vi "Async.Engine.Close.vi"(8 "error in (no error)":errorcluster, 11 "Async in":refnum<class "VS Inline Async API.lvclass">) -> (0 "error out":errorcluster, 3 "Async out":refnum<class "VS Inline Async API.lvclass">)   [LabVIEW 2015, in "VS Inline Async API.lvlib" / "VS Inline Async API.lvclass"]
uses:
  VS Inline Async API.lvclass
  VS Inline Async API.lvclass/VS Inline Async API.ctl
  <vilib>/NI Veristand/Custom Device Tools/Custom Device Utility Library/NI VeriStand - Print Debug String.vi
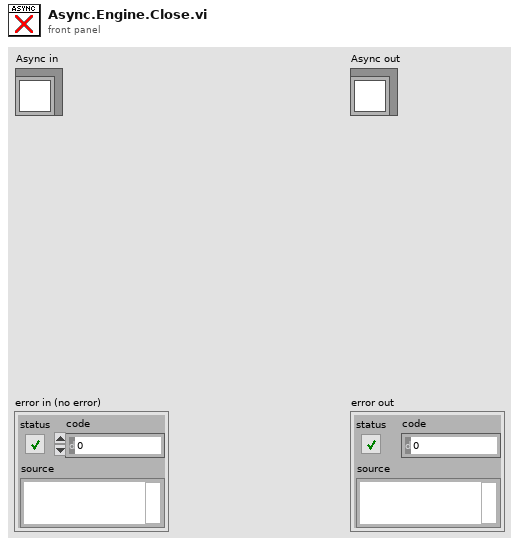
[diagram p1: front panel]
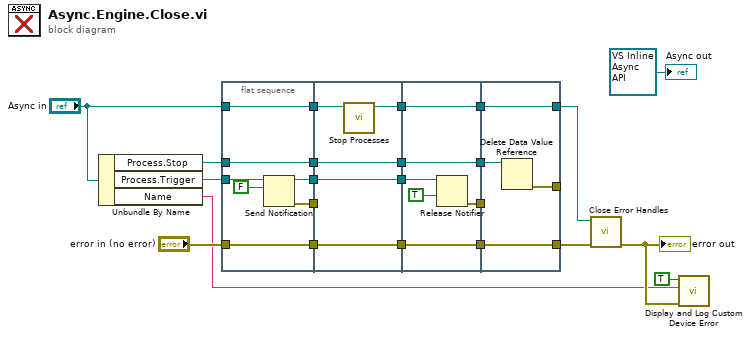
[diagram p0: block diagram]
diagram:
  n1 = Unbundle By Name("Async in") -> ("Process.Stop"=w9:refnum<data-value>, "Process.Trigger"=w16:refnum<notifier>, "Name"=w12:string)
  n2 = flat-sequence {
    tunnel: [w30] -> w23
    tunnel: "error in (no error)" -> [w30]
    tunnel: [w28] -> w19
    tunnel: [w27] -> w17
    tunnel: w16 -> [w26]
    tunnel: [w25] -> w11
    tunnel: "Async in" -> [w25]
    tunnel: w9 -> [w24]
    tunnel: [w24] -> w6
    tunnel: [w35] -> w22
    tunnel: w23 -> [w35]
    tunnel: w19 -> [_]
    tunnel: [w34] -> w18
    tunnel: w17 -> [w34]
    tunnel: w11 -> [w33]
    tunnel: [w32] -> w7
    tunnel: w6 -> [w32]
    tunnel: [w31] -> w4
    tunnel: w22 -> [w41]
    tunnel: w18 -> [w39]
    tunnel: [w41] -> w10
    tunnel: [w38] -> w8
    tunnel: w7 -> [w38]
    tunnel: [w37] -> w5
    tunnel: w4 -> [w37]
    tunnel: [w36] -> w1
    tunnel: [w45] -> w20
    tunnel: w10 -> [w45]
    tunnel: w8 -> [w44]
    tunnel: [w43] -> w2
    tunnel: w5 -> [w43]
    tunnel: w1 -> [_]
    tunnel: [w42] -> _
    frame #0 {
      n3 = Send Notification(notification=FALSE, notifier=w26) -> (notifier out=w27:refnum<notifier>, error out=w28:errorcluster)  [unwired: 1 in]
    }
    frame #1 {
      n4 = call "Stop Processes.vi"("VS Inline Async API in"=w33) -> ("VS Inline Async API out"=w31:refnum<class "VS Inline Async API.lvclass">)  [unwired: 10 in]
    }
    frame #2 {
      n5 = Release Notifier(notifier=w39, force destroy? (F)=TRUE ("notification")) -> (error out=w36:errorcluster)  [unwired: 1 in, 2 out]
    }
    frame #3 {
      n6 = Delete Data Value Reference(data value reference=w44) -> (error out=w42:errorcluster)  [unwired: 1 in, 1 out]
    }
  }
  n7 = call "Close Error Handles.vi"("error in"=w20, "Async in"=w2) -> ("error out"=w14:errorcluster)  [unwired: 8 in, 1 out]
  "error out" <- w14
  n8 = call "Display and Log Custom Device Error.vi"("error out"=w14, "Your code's public name"=w12, "Custom Device? (T)"=TRUE) -> ()  [unwired: 9 in]
  "Async out" <- refnum<class "VS Inline Async API.lvclass"> refnum ("Async out")
